vi "Custom Error Cfg Path.vi"(8 "error in (no error)":errorcluster) -> (0 "error out":errorcluster, 3 "path":path)   [LabVIEW 2026, in "PXI_Common.lvlib"]
uses:
  PXI_Common.lvlib
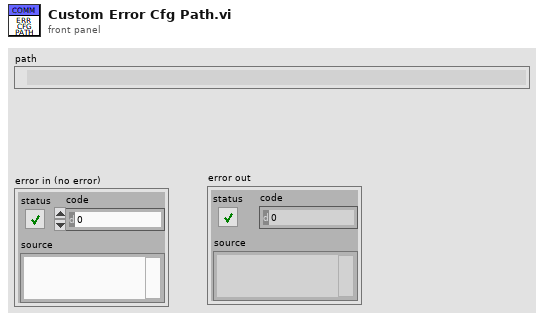
[diagram p1: front panel]
types:
  T1 = enum32{"invalid app kind", "Development System", "Run Time System", "Student Edition", "Embedded LabVIEW", "Evaluation", "Custom"}
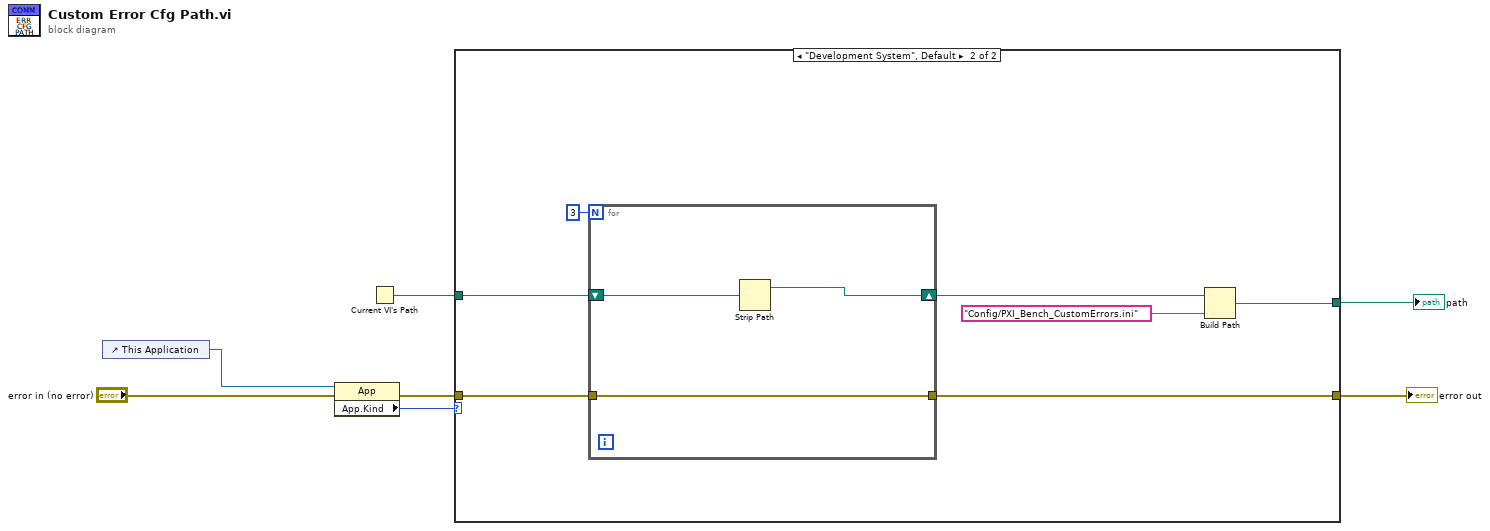
[diagram p0: block diagram]
diagram:
  n1 = control-ref of="This Application"() -> (w6:refnum<vi>)
  n2 = property class="App"(reference=w6, error in="error in (no error)") -> (error out=w4:errorcluster, "App.Kind"=w5:T1)  [unwired: 1 out]
  n3 = Current VI's Path() -> (path=w3:path)
  n4 = case shown="\"Development System\", Default" w5 {
    tunnel: w4 -> [w9 w16]
    tunnel: w3 -> [w8 w15]
    tunnel: [w8 w11] -> w2
    tunnel: [w9 w14] -> w1
    frame "Run Time System" {
    }
    frame "Development System", Default {
      n5 = for {
        N: 3 -> [_]
        tunnel: w16 -> [w18]
        tunnel: [w18] -> w14
        shift-right: [w17] -> w12
        shift-left: w15 -> [w19]
        n6 = Strip Path(path=w19) -> (stripped path=w17:path)  [unwired: 1 out]
      }
      n7 = Build Path(base path=w12, name or relative path="Config/PXI_Bench_CustomErrors.ini") -> (appended path=w11:path)
    }
  }
  "error out" <- w1
  "path" <- w2
